vi "Enable Output.vi"(8 "error in (no error)":errorcluster, 10 "Enable Output  (T: Enable)":bool=TRUE, 11 "VISA resource name":refnum<visa-resource-name>) -> (0 "error out":errorcluster, 3 "VISA resource name out":refnum<visa-resource-name>)   [LabVIEW 2013, in "AWG.lvlib" / "Agilent 33XXX Series.lvlib"]
doc: "Enables or disables the output connector.\n\n<B>Note:</B> This functionality is not supported on the 33120 model. This VI will not perform any instrument communication with the 33120."
uses:
  Agilent 33XXX Series.lvlib
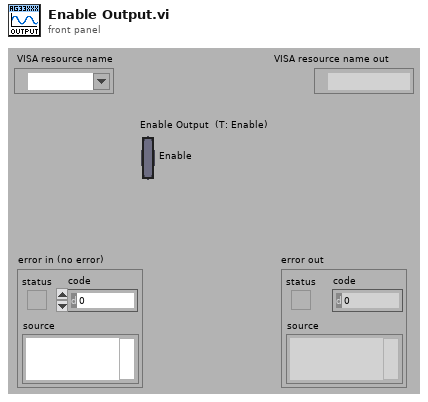
[diagram p1: front panel]
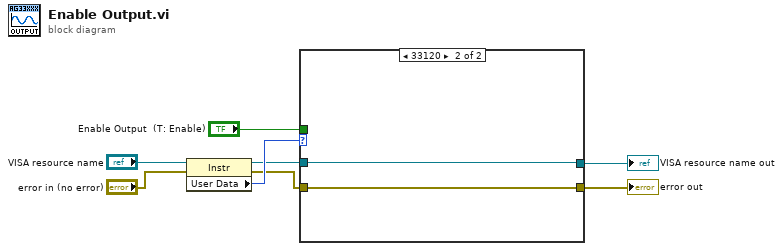
[diagram p0: block diagram]
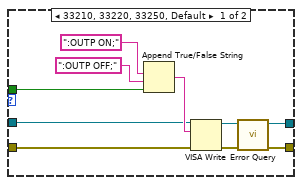
[diagram p2: hidden frame]
diagram:
  n1 = property on="Property Node" class="Instr"(reference="VISA resource name", error in="error in (no error)") -> (reference out=w7:refnum<visa-resource-name>, error out=w6:errorcluster, "User Data"=w8:u32)
  n2 = case shown="33120" w8 {
    tunnel: [w13 w20] -> w3
    tunnel: [w12 w19] -> w4
    tunnel: w7 -> [w11 w20]
    tunnel: w6 -> [w10 w19]
    tunnel: "Enable Output  (T: Enable)" -> [w9 _]
    frame 33210, 33220, 33250, Default {
      n3 = Append True/False String(1:w9, 2:":OUTP OFF;" ("true string"), 3:":OUTP ON;" ("true string")) -> (0:w16:string)  [unwired: 1 in]
      n4 = VISA Write(VISA resource name=w11, write buffer=w16, error in (no error)=w10) -> (VISA resource name out=w14:refnum<visa-resource-name>, error out=w15:errorcluster)  [unwired: 1 out]
      n5 = call "Error Query.vi"("error in (no error)"=w15, "VISA resource name"=w14) -> ("error out"=w12:errorcluster, "VISA resource name out"=w13:refnum<visa-resource-name>)  [unwired: 6 in, 2 out]
    }
    frame 33120 {
    }
  }
  "error out" <- w4
  "VISA resource name out" <- w3
